vi "App.Save.vi"(8 "error in (no error)":errorcluster, 11 "State Variables":T1) -> (0 "error out":errorcluster)   [LabVIEW 2013, in "Simple Sequence Editor.lvlib"]
uses:
  Simple Sequence Editor.lvlib
  Types/StateVariables.ctl
  Types/ChannelProperties.ctl
  Types/Saved.Sequence.ctl
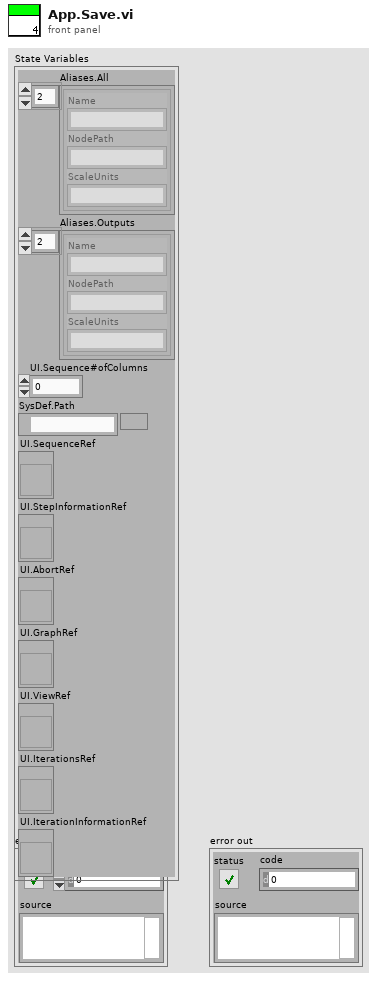
[diagram p1: front panel]
types:
  T1 = typedef "Simple Sequence Editor.lvlib/StateVariables.ctl" = cluster{"Aliases.All":T2[], "Aliases.Outputs":T2[], "UI.Sequence#ofColumns":i32, "SysDef.Path":path, "UI.SequenceRef":refnum<vi>, "UI.StepInformationRef":refnum<vi>, "UI.AbortRef":refnum<vi>, "UI.GraphRef":refnum<vi>, "UI.ViewRef":refnum<vi>, "UI.IterationsRef":refnum<vi>, "UI.IterationInformationRef":refnum<vi>}
  T2 = typedef "Simple Sequence Editor.lvlib/ChannelProperties.ctl" = cluster{"Name":string, "NodePath":string, "ScaleUnits":string}
  T3 = typedef "Simple Sequence Editor.lvlib/Saved.Sequence.ctl" = cluster{"Output Channels":T2[], "Item Names":string[][], "Step":string, "Abort":string, "Iterations":u32, "Iteration":string}
  T4 = enum16{"open", "replace", "create", "open or create", "replace or create", "replace or create with confirmation"}
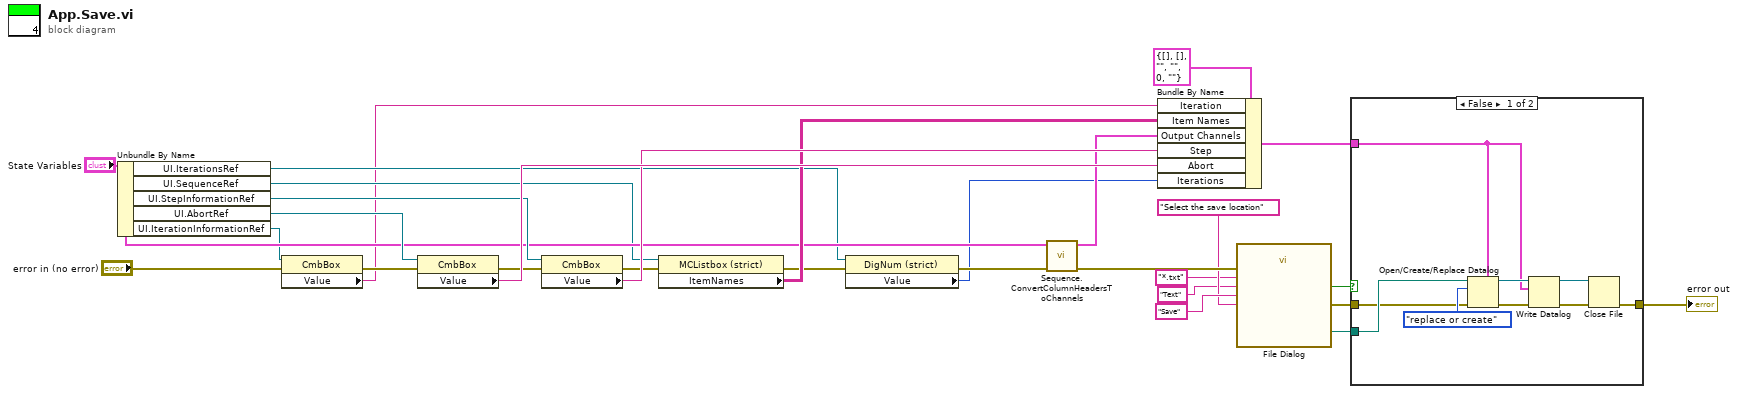
[diagram p0: block diagram]
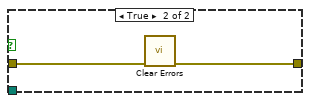
[diagram p2: hidden frame]
diagram:
  n1 = Unbundle By Name("State Variables") -> ("UI.IterationsRef"=w8:refnum<vi>, "UI.SequenceRef"=w9:refnum<vi>, "UI.StepInformationRef"=w20:refnum<vi>, "UI.AbortRef"=w21:refnum<vi>, "UI.IterationInformationRef"=w4:refnum<vi>)
  n2 = property class="CmbBox"(reference=w4, error in="error in (no error)") -> (error out=w2:errorcluster, "Value"=w1:string)  [unwired: 1 out]
  n3 = property class="CmbBox"(reference=w21, error in=w2) -> (error out=w22:errorcluster, "Value"=w28:string)  [unwired: 1 out]
  n4 = property class="CmbBox"(reference=w20, error in=w22) -> (error out=w23:errorcluster, "Value"=w27:string)  [unwired: 1 out]
  n5 = property class="MCListbox (strict)"(reference=w9, error in=w23) -> (error out=w7:errorcluster, "ItemNames"=w26:string[][])  [unwired: 1 out]
  n6 = property class="DigNum (strict)"(reference=w8, error in=w7) -> (error out=w6:errorcluster, "Value"=w5:u32)  [unwired: 1 out]
  n7 = call "Sequence.ConvertColumnHeadersToChannels.vi"("error in (no error)"=w6, "State Variables"="State Variables") -> ("error out"=w19:errorcluster, "Output Channels"=w25:T2[])  [unwired: 8 in]
  n8 = Bundle By Name(cluster=T3 {"Output Channels"=[], "Item Names"=[], "Step"="", "Abort"="", "Iterations"=0, "Iteration"=""}, "Iteration"=w1, "Item Names"=w26, "Output Channels"=w25, "Step"=w27, "Abort"=w28, "Iterations"=w5) -> (w29:T3)
  n9 = call "File Dialog"("prompt"="Select the save location", "button label"="Save", "error in"=w19, "pattern (all files)"="*.txt", "pattern label"="Text") -> ("selected path"=w15:path, "cancelled"=w16:bool, "error out"=w11:errorcluster)  [unwired: 7 in, 1 out]
  n10 = case shown="False" w16 {
    tunnel: [w38 w39] -> w10
    tunnel: w11 -> [w35 w40]
    tunnel: w15 -> [w37 _]
    tunnel: w29 -> [w31 _]
    frame False {
      n11 = Open/Create/Replace Datalog(5:w31, 8:w35, 10:T4."replace or create" ("operation (0:open)"), 11:w37) -> (0:w34:errorcluster, 3:w32:refnum<k1>)  [unwired: 2 in, 1 out]
      n12 = Write Datalog(4:w34, 6:w31, 7:w32) -> (0:w33:errorcluster, 3:w30:refnum<k1>)
      n13 = Close File(refnum=w30, error in=w33) -> (error out=w38:errorcluster)  [unwired: 1 out]
    }
    frame True {
      n14 = call <vilib>:"Clear Errors.vi"("error in (no error)"=w40) -> ("error out"=w39:errorcluster)  [unwired: 6 in]
    }
  }
  "error out" <- w10
